vi "DQtoAlphaBeta_noSine.vi"(0 "direct":sgl format="%#_30g", 1 "cosx":sgl, 2 "sinx":sgl, 5 "quadrature":sgl format="%#_30g", 12 "Resources":T1) -> (4 "alpha":sgl format="%#_30g", 6 "beta":sgl format="%#_30g")   [LabVIEW 2017]
uses:
  Multiplier/Multiplier.lvclass
  Adder/Adder.lvclass
  Subtractor/Subtractor.lvclass
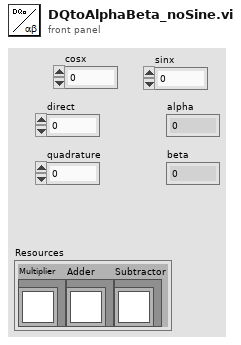
[diagram p1: front panel]
types:
  T1 = cluster{"Multiplier":refnum<class "Multiplier.lvclass">, "Adder":refnum<class "Adder.lvclass">, "Subtractor":refnum<class "Subtractor.lvclass">}
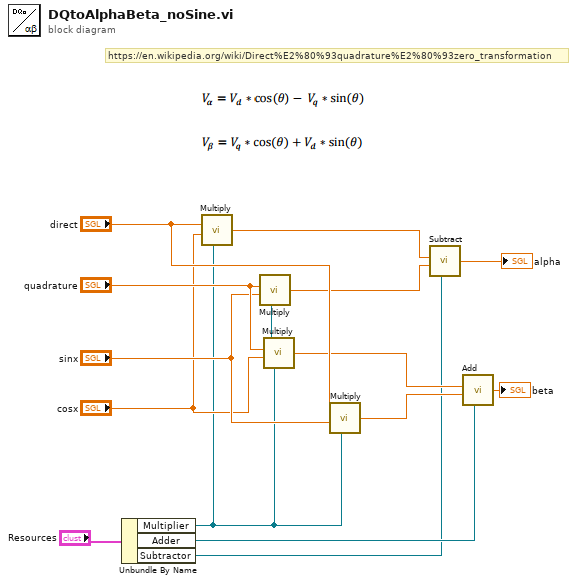
[diagram p0: block diagram]
diagram:
  # "https://en.wikipedia.org/wiki/Direct%E2%80%93quadrature%E2%80%93zero_transformation"
  n1 = Unbundle By Name("Resources") -> ("Multiplier"=w9:refnum<class "Multiplier.lvclass">, "Adder"=w2:refnum<class "Adder.lvclass">, "Subtractor"=w1:refnum<class "Subtractor.lvclass">)
  n2 = call-dynamic "Multiply.vi"("x"="direct", "y"="cosx", "Multiplier"=w9) -> ("x*y"=w8:sgl)  [unwired: 4 in]
  n3 = call-dynamic "Multiply.vi"("x"="quadrature", "y"="sinx", "Multiplier"=w9) -> ("x*y"=w7:sgl)  [unwired: 4 in]
  n4 = call-dynamic "Multiply.vi"("x"="quadrature", "y"="cosx", "Multiplier"=w9) -> ("x*y"=w5:sgl)  [unwired: 4 in]
  n5 = call-dynamic "Multiply.vi"("x"="direct", "y"="sinx", "Multiplier"=w9) -> ("x*y"=w4:sgl)  [unwired: 4 in]
  n6 = call-dynamic "Subtract.vi"("x"=w8, "y"=w7, "Subtractor"=w1) -> ("x-y"=→"alpha":sgl)  [unwired: 4 in]
  n7 = call-dynamic "Add.vi"("x"=w5, "y"=w4, "Adder"=w2) -> ("x+y"=→"beta":sgl)  [unwired: 4 in]
